vi "FTW-CodeGen-GenerateCode.vi"(0 "State In":T2, 5 "XRef":refnum<vi>, 7 "Terms":T1(array[cluster]), 9 "Diagram":refnum<vi>) -> (4 "State Out":T2, 6 "Reply":string[](array[string]), 8 "Generated Code?":bool)   [LabVIEW 2012, in "FTW-JSON-Deserialize.xnode"]
uses:
  FTW-JSON-Deserialize.xnode
  FTW-CodeGen-State.ctl
  FTW-CodeGen-Prototype.vi
panel:
  # "Inputs"
  # "Outputs"
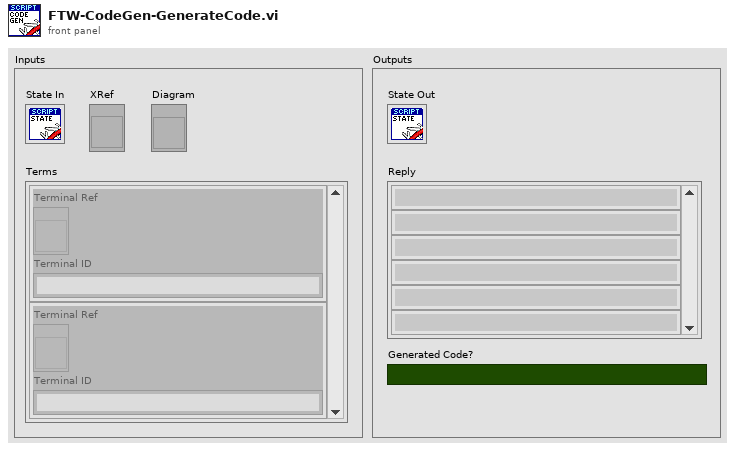
[diagram p1: front panel]
types:
  T1 = cluster{"Terminal Ref":refnum<vi>, "Terminal ID":string}[]
  T2 = typedef "FTW-JSON-Deserialize.xnode/FTW-CodeGen-State.ctl" = cluster{"Dummy":string}
  T3 = typedef "LVPositionTypeDef.ctl" = cluster{"Left":i32, "Top":i32}
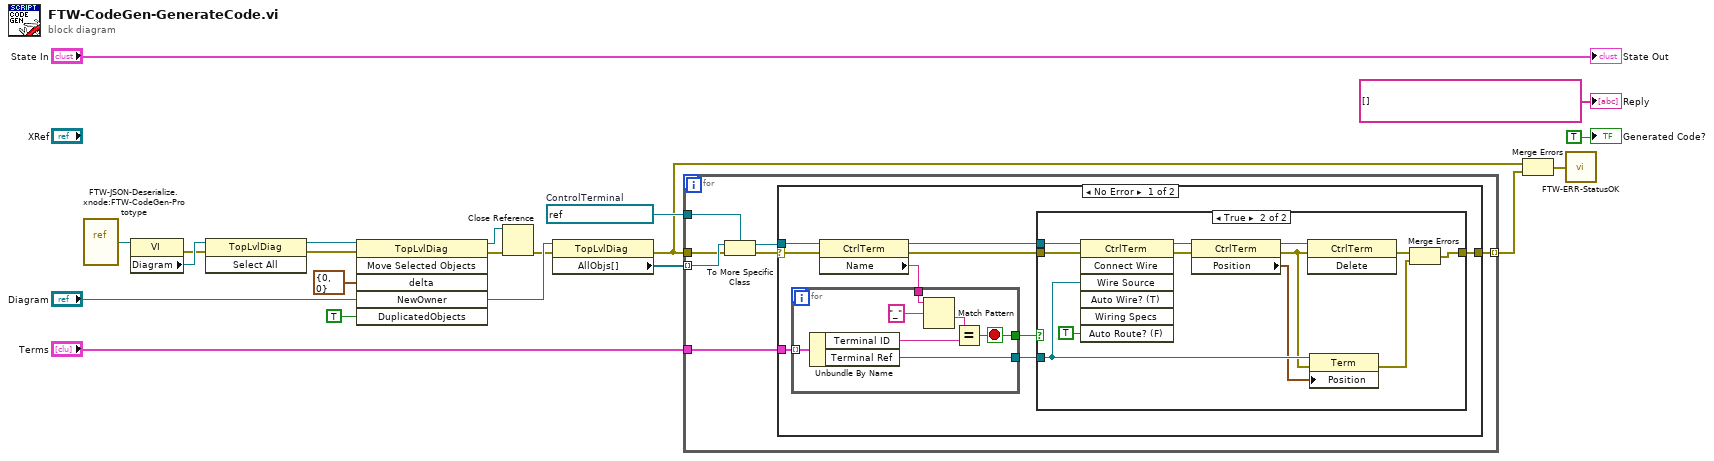
[diagram p0: block diagram]
diagram:
  w15 = refnum<vi> refnum  # ControlTerminal
  n1 = vi-ref "FTW-JSON-Deserialize.xnode:FTW-CodeGen-Prototype.vi"() -> (w5:refnum<vi>)
  n2 = property class="VI"(reference=w5) -> (error out=w4:errorcluster, "Diagram"=w14:refnum<vi>)  [unwired: 1 in, 1 out]
  n3 = invoke class="TopLvlDiag" method="Select All"(reference=w14, error in=w4) -> (reference out=w18:refnum<vi>, error out=w17:errorcluster)  [unwired: 1 in, 1 out]
  n4 = invoke class="TopLvlDiag" method="Move Selected Objects"(reference=w18, error in=w17, "delta"=cluster{"X":i32, "Y":i32} {"X"=0, "Y"=0} ("X/Y Delta"), "NewOwner"="Diagram", "DuplicatedObjects"=TRUE ("Duplicate? (F)")) -> (reference out=w3:refnum<vi>, error out=w2:errorcluster)  [unwired: 1 in, 4 out]
  n5 = Close Reference(reference=w3, error in (no error)=w2) -> (error out=w1:errorcluster)
  n6 = property class="TopLvlDiag"(reference="Diagram", error in=w1) -> (error out=w12:errorcluster, "AllObjs[]"=w16:refnum<vi>[])  [unwired: 1 out]
  n7 = for {
    tunnel: w16 -> [w27] mode=indexing
    tunnel: w12 -> [w26]
    tunnel: w15 -> [w25]
    tunnel: "Terms" -> [w22]
    tunnel: [w21] -> w13 mode=indexing
    n8 = To More Specific Class(target class=w25, reference=w27, error in=w26) -> (specific class reference=w23:refnum<vi>, error out=w24:errorcluster)
    n9 = case shown="No Error" w24 {
      selector: w24 -> [w35 _]
      tunnel: w23 -> [w36 _]
      tunnel: w22 -> [w34 _]
      tunnel: [w29 _] -> w21
      frame No Error {
        n10 = property class="CtrlTerm"(reference=w36, error in=w35) -> (reference out=w31:refnum<vi>, error out=w30:errorcluster, "Name"=w33:string)
        n11 = for {
          tunnel: w34 -> [w56] mode=indexing
          tunnel: w33 -> [w54]
          tunnel: [w55] -> w32
          tunnel: [w50] -> w28
          stop <- w50 stop-if-true
          n12 = Unbundle By Name(w56) -> ("Terminal ID"=w51:string, "Terminal Ref"=w55:refnum<vi>)
          n13 = Match Pattern(string=w54, regular expression="_") -> (after substring=w52:string)  [unwired: 1 in, 3 out]
          n14 = Equal?(x=w52, y=w51) -> (x = y?=w50:bool)
        }
        n15 = case shown="True" w28 {
          tunnel: w32 -> [_ w41]
          tunnel: w31 -> [_ w49]
          tunnel: w30 -> [w37 w48]
          tunnel: [w37 w43] -> w29
          frame False {
          }
          frame True {
            n16 = invoke class="CtrlTerm" method="Connect Wire"(reference=w49, error in=w48, "Wire Source"=w41, "Auto Route? (F)"=TRUE) -> (reference out=w47:refnum<vi>, error out=w45:errorcluster)  [unwired: 3 in, 5 out]
            n17 = property class="CtrlTerm"(reference=w47, error in=w45) -> (reference out=w46:refnum<vi>, error out=w40:errorcluster, "Position"=w38:T3)
            n18 = invoke class="CtrlTerm" method="Delete"(reference=w46, error in=w40) -> (error out=w44:errorcluster)  [unwired: 1 in, 2 out]
            n19 = property class="Term"(reference=w41, error in=w40, "Position"=w38) -> (error out=w39:errorcluster)  [unwired: 1 out]
            n20 = Merge Errors(w44, w39) -> (w43:errorcluster)
          }
        }
      }
      frame Error {
      }
    }
  }
  n21 = Merge Errors(w12, w13) -> (w10:errorcluster)
  n22 = call "FTW-ERR-StatusOK.vi"("error to check"=w10) -> ()  [unwired: 1 out]
  "State Out" <- "State In"
  "Reply" <- string[] [] ("Reply")
  "Generated Code?" <- TRUE ("Generated Code?")
